vi "Read Data.vi"(8 "error in (no error)":errorcluster, 11 "CRDS in":refnum<class "CRDS.lvclass">=refnum) -> (0 "error out":errorcluster, 2 "CRDS":refnum<class "CRDS Data.lvclass">, 3 "CRDS out":refnum<class "CRDS.lvclass">)   [LabVIEW 2014, in "CRDS.lvclass"]
uses:
  CRDS.lvclass
  Data/Main/CRDS Data.lvclass
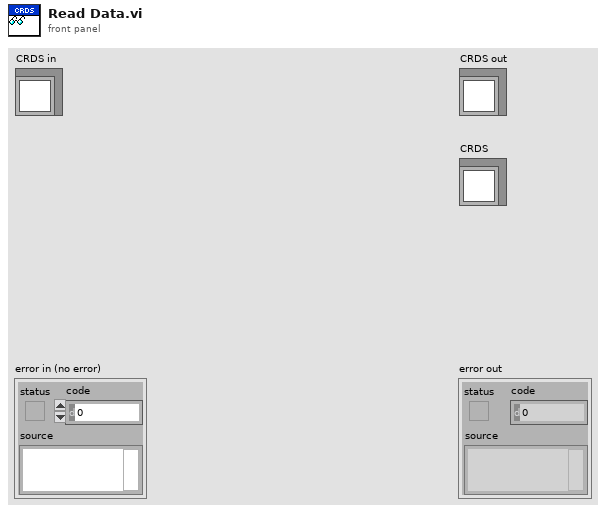
[diagram p1: front panel]
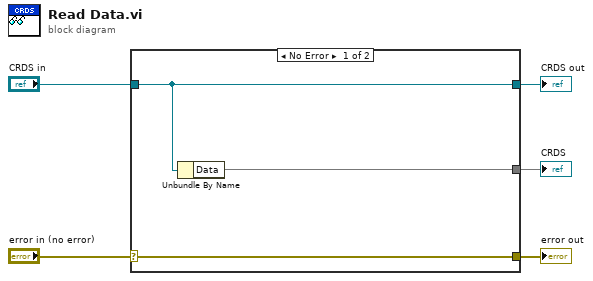
[diagram p0: block diagram]
diagram:
  n1 = case shown="No Error" "error in (no error)" {
    selector: "error in (no error)" -> [w8 w9]
    tunnel: [w8 w9] -> w4
    tunnel: [w7 w10] -> w2
    tunnel: "CRDS in" -> [w7 w10]
    tunnel: [w6 _] -> w1
    frame No Error {
      n2 = Unbundle By Name(w7) -> ("Data"=w6)
    }
    frame Error {
    }
  }
  "error out" <- w4
  "CRDS out" <- w2
  "CRDS" <- w1
